vi "data-Write.vi"(6 "Reject New Tag(F)":bool, 8 "error in (no error)":errorcluster, 9 "Value":variant, 10 "name":string, 11 "Cluster in":T1) -> (0 "error out":errorcluster, 2 "Created":bool, 3 "Cluster out":T1)   [LabVIEW 2017, in "TagDB.lvlib"]
uses:
  TagDB.lvlib
  Typedef/tagdb-data.ctl
  <vilib>/Utility/Data Type/NI_Data Type.lvlib
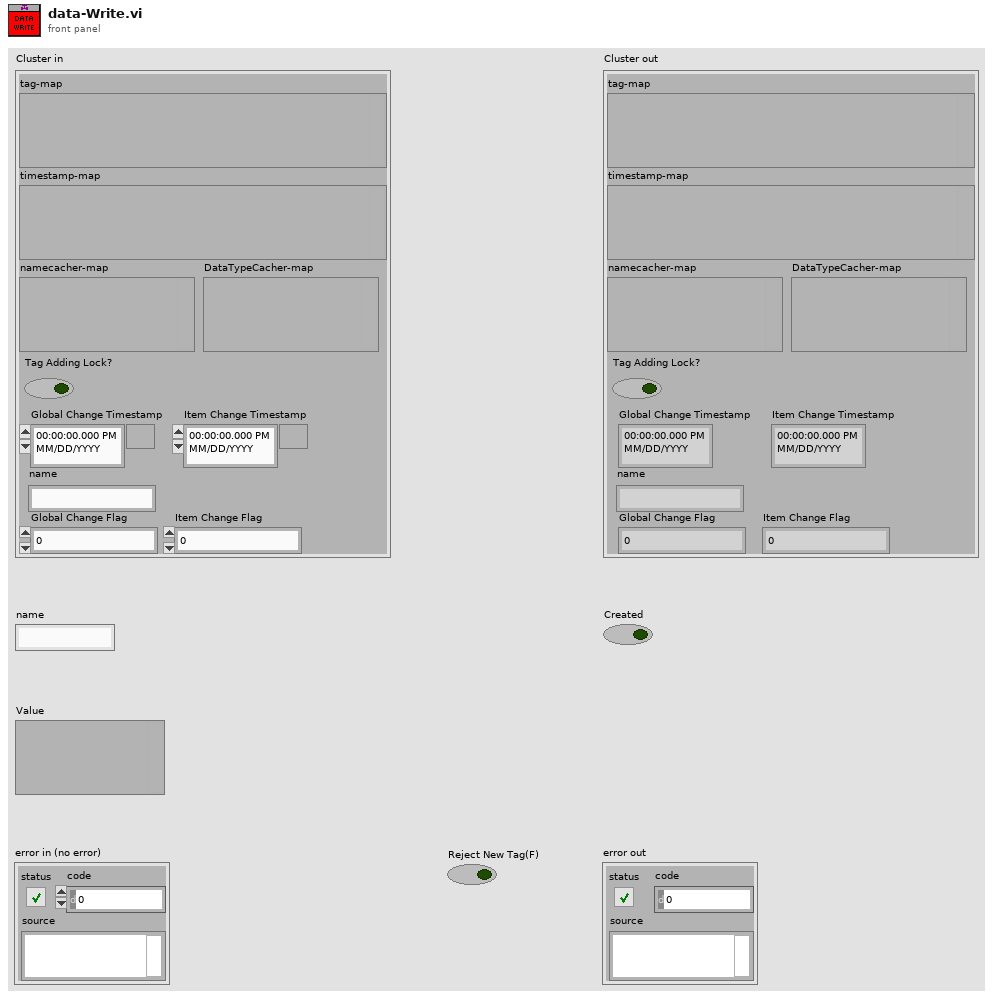
[diagram p1: front panel]
types:
  T1 = typedef "TagDB.lvlib/tagdb-data.ctl" = cluster{"tag-map":variant, "timestamp-map":variant, "namecacher-map":variant, "DataTypeCacher-map":variant, "Tag Adding Lock?":bool, "Global Change Timestamp":timestamp, "Item Change Timestamp":timestamp, "name":string, "Global Change Flag":u64, "Item Change Flag":u64}
  T2 = typedef "NI_Data Type.lvlib/Data Type.ctl" = enum8{"Invalid Type", "Void", "I8", "I16", "I32", "I64", "U8", "U16", "U32", "U64", "Single Float", "Double Float", "Extended Float", "Single Complex", "Double Complex", "Extended Complex", "Enum U8", "Enum U16", "Enum U32", "Enum U64", "Single Float With Unit", "Double Float With Unit", "Extended Float With Unit", "Single Complex with Unit", "Double Complex with Unit", "Extended Complex with Unit", "Boolean", "String", "Path", "Picture", "Tag", "Array", "Cluster", "Variant", "LV Variant", "Waveform", "Timestamp", "Digital Waveform", "Digital Data", "ExpressData", "Refnum", "External Data", "VI", "Poly VI", "LabVIEW Class Instance", "Fixed Point"}
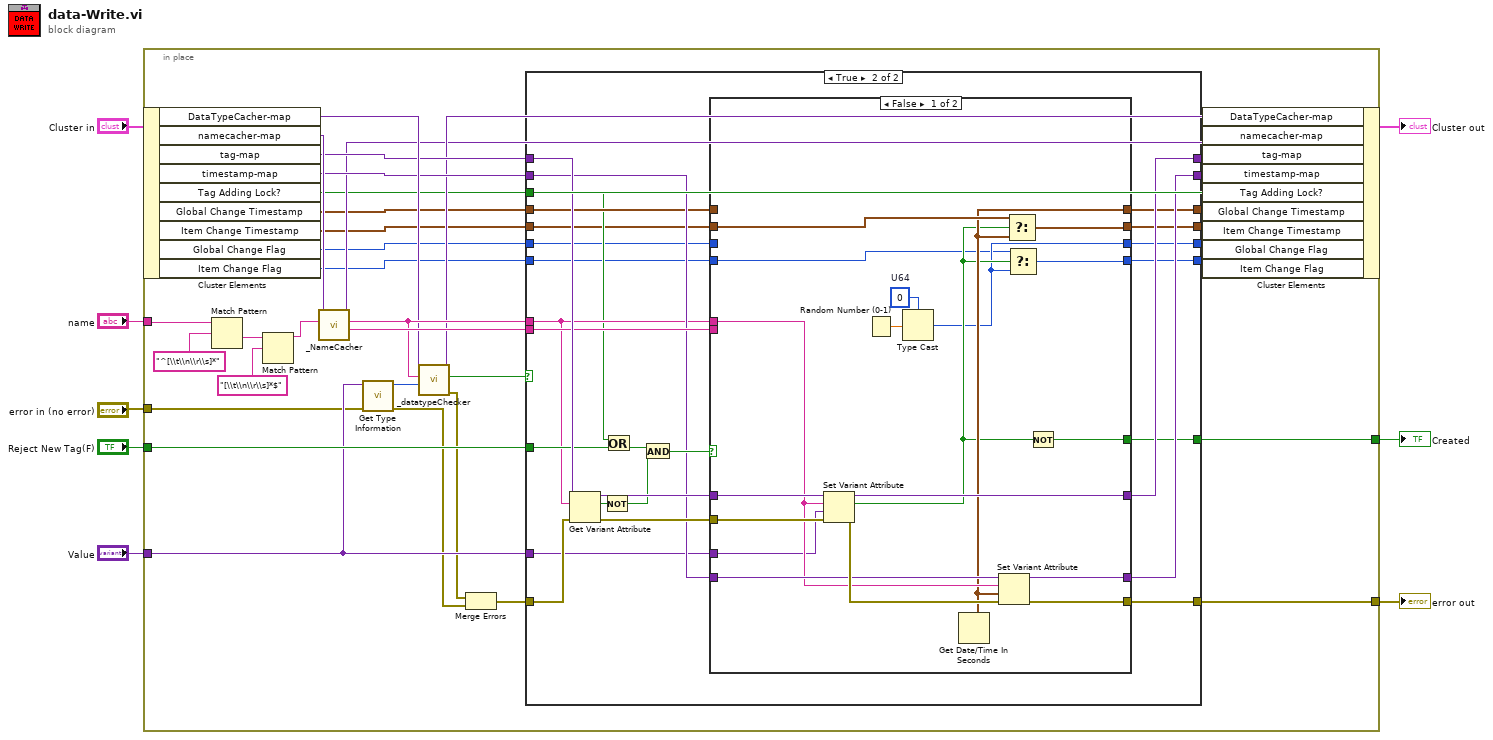
[diagram p0: block diagram]
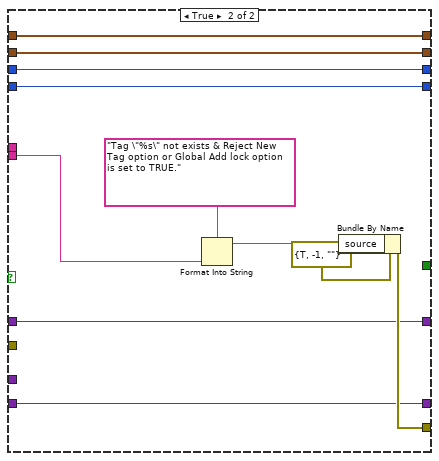
[diagram p3: hidden frame]
diagram:
  n1 = in-place "In Place Element Structure" {
    in-place-border: [w42] -> w1
    in-place-border: "Reject New Tag(F)" -> [w41]
    in-place-border: "name" -> [w10]
    in-place-border: "Value" -> [w38]
    in-place-border: "error in (no error)" -> [w24]
    in-place-border: [w18] -> w8
    n2 = in-place-cluster #1("Cluster in") -> ("DataTypeCacher-map"=w34:variant, "namecacher-map"=w33:variant, "tag-map"=w32:variant, "timestamp-map"=w31:variant, "Tag Adding Lock?"=w21:bool, "Global Change Timestamp"=w23:timestamp, "Item Change Timestamp"=w20:timestamp, "Global Change Flag"=w16:u64, "Item Change Flag"=w15:u64)
    n3 = Match Pattern(string=w10, regular expression="^[\\t\\n\\r\\s]*") -> (after substring=w13:string)  [unwired: 1 in, 3 out]
    n4 = Match Pattern(string=w13, regular expression="[\\t\\n\\r\\s]*$") -> (before substring=w9:string)  [unwired: 1 in, 3 out]
    n5 = call "_NameCacher.vi"("key"=w9, "cacher"=w33) -> ("Raw name"=w40:string, "Key in lower case"=w39:string, "cacher out"=w29:variant)  [unwired: 7 in]
    n6 = call <vilib>:"Get Type Information.vi"("error in (no error)"=w24, "Variant"=w38) -> ("error out"=w26:errorcluster, "Type"=w37:T2)  [unwired: 5 in, 3 out]
    n7 = call "_datatypeChecker.vi"("Type"=w37, "key"=w39, "cacher (in)"=w34) -> ("error out"=w25:errorcluster, "match?"=w35:bool, "cacher"=w30:variant)  [unwired: 5 in, 1 out]
    n8 = Merge Errors(w25, w26) -> (w36:errorcluster)
    n9 = case shown="True" w35 {
      tunnel: w32 -> [w48 w75]
      tunnel: w31 -> [w47 w65]
      tunnel: [w49 w74] -> w42
      tunnel: w41 -> [_ w73]
      tunnel: w40 -> [_ w71]
      tunnel: w39 -> [_ w63]
      tunnel: w38 -> [_ w62]
      tunnel: w36 -> [w49 w70]
      tunnel: [w48 w66] -> w28
      tunnel: [w47 w64] -> w27
      tunnel: w23 -> [w46 w60]
      tunnel: [w46 w61] -> w22
      tunnel: w21 -> [_ w58]
      tunnel: w20 -> [w45 w56]
      tunnel: [w45 w57] -> w19
      tunnel: [_ w54] -> w18
      tunnel: [w44 w53] -> w17
      tunnel: w16 -> [w44 w52]
      tunnel: w15 -> [w43 w51]
      tunnel: [w43 w50] -> w14
      frame False {
      }
      frame True {
        n10 = Get Variant Attribute(Variant=w75, name=w63, error in=w70) -> (duplicate Variant=w67:variant, found=w69:bool, error out=w68:errorcluster)  [unwired: 1 in, 1 out]
        n11 = Not(x=w69) -> (.not. x?=w55:bool)
        n12 = Or(x=w58, y=w73) -> (x .or. y?=w59:bool)
        n13 = And(x=w59, y=w55) -> (x .and. y?=w72:bool)
        n14 = case shown="False" w72 {
          tunnel: [w93 w102] -> w74
          tunnel: w71 -> [_ w103]
          tunnel: w68 -> [w92 _]
          tunnel: w67 -> [w91 w100]
          tunnel: [w90 w100] -> w66
          tunnel: w65 -> [w89 w99]
          tunnel: [w88 w99] -> w64
          tunnel: w63 -> [w87 _]
          tunnel: w62 -> [w86 _]
          tunnel: [w84 w98] -> w61
          tunnel: w60 -> [_ w98]
          tunnel: [w83 w97] -> w57
          tunnel: w56 -> [w85 w97]
          tunnel: [w82 _] -> w54
          tunnel: [w77 w96] -> w53
          tunnel: w52 -> [_ w96]
          tunnel: w51 -> [w76 w95]
          tunnel: [w78 w95] -> w50
          frame False {
            w80 = u64 0  # U64
            n15 = Set Variant Attribute(Variant=w91, name=w87, value=w86, error in=w92) -> (Variant out=w90:variant, replaced=w79:bool, error out=w94:errorcluster)
            n16 = Random Number (0-1)() -> (number: 0 to 1=w81:dbl)
            n17 = Type Cast(type=w80, x=w81) -> (*(type *) &x=w77:u64)
            n18 = Get Date/Time In Seconds() -> (seconds since 1Jan1904=w84:timestamp)
            n19 = Set Variant Attribute(Variant=w89, name=w87, value=w84, error in=w94) -> (Variant out=w88:variant, error out=w93:errorcluster)  [unwired: 1 out]
            n20 = Select(t=w85, s=w79, f=w84) -> (s? t:f=w83:timestamp)
            n21 = Select(t=w76, s=w79, f=w77) -> (s? t:f=w78:u64)
            n22 = Not(x=w79) -> (.not. x?=w82:bool)
          }
          frame True {
            n23 = Format Into String(format string="Tag \"%s\" not exists & Reject New Tag option or Global Add lock option is set to TRUE." ("source"), w103) -> (resulting string=w101:string)  [unwired: 2 in, 1 out]
            n24 = Bundle By Name(cluster=errorcluster {"status"=TRUE, "code"=-1, "source"=""} ("error IO"), "source"=w101) -> (w102:errorcluster)
          }
        }
      }
    }
    n25 = in-place-cluster #1("DataTypeCacher-map"=w30, "namecacher-map"=w29, "tag-map"=w28, "timestamp-map"=w27, "Tag Adding Lock?"=w21, "Global Change Timestamp"=w22, "Item Change Timestamp"=w19, "Global Change Flag"=w17, "Item Change Flag"=w14) -> (→"Cluster out":T1)
  }
  "Created" <- w8
  "error out" <- w1
